vi "Percent-Decode String.vi"(10 "Pct-Encoded String":string) -> (2 "String":string)   [LabVIEW 2013, in "openURI.lvlib"]
uses:
  openURI.lvlib
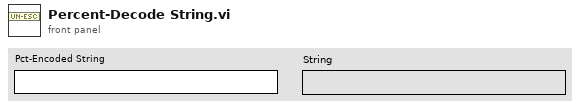
[diagram p1: front panel]
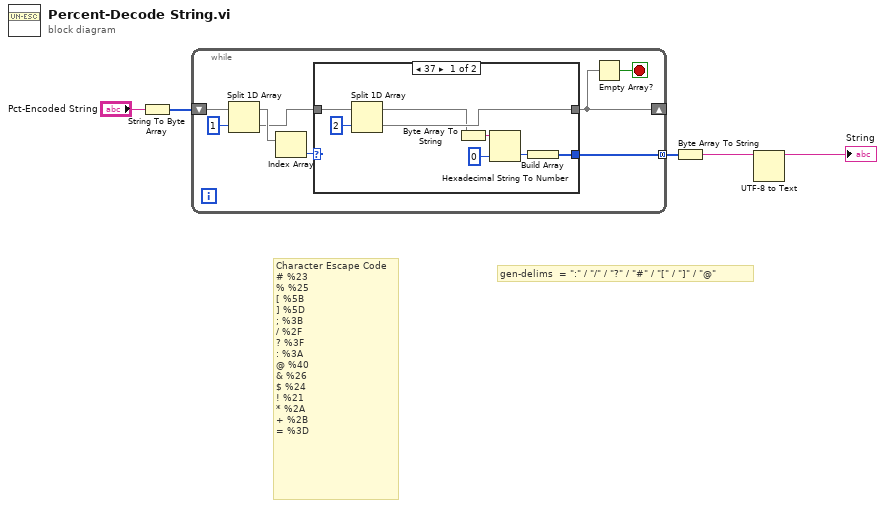
[diagram p0: block diagram]
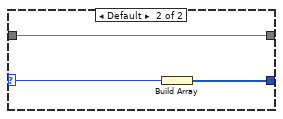
[diagram p2: hidden frame]
diagram:
  # "gen-delims  = \":\" / \"/\" / \"?\" / \"#\" / \"[\" / \"]\" / \"@\""
  # "Character\tEscape Code\n#\t%23\n%\t%25\n[\t%5B\n]\t%5D\n;\t%3B\n/\t%2F\n?\t%3F\n:\t%3A\n@\t%40\n&\t%26\n$\t%24\n!\t%21\n*\t%2A\n+\t%2B\n=\t%3D"
  n1 = String To Byte Array(string="Pct-Encoded String") -> (unsigned byte array=w5:u8[])
  n2 = while {
    shift-right: [w6] -> _
    shift-left: w5 -> [w13]
    tunnel: [w7] -> w4 mode=concatenating
    stop <- w10 stop-if-true
    n3 = Split 1D Array(array=w13, index=1) -> (first subarray=w11:u8[], second subarray=w8:u8[])
    n4 = Index Array(array=w11) -> (element=w9:u8)  [unwired: 1 in]
    n5 = case shown="37" w9 {
      selector: w9 -> [_ w23]
      tunnel: w8 -> [w20 w24]
      tunnel: [w19 w24] -> w6
      tunnel: [w15 w22] -> w7
      frame 37 {
        n6 = Split 1D Array(array=w20, index=2) -> (first subarray=w18:u8[], second subarray=w19:u8[])
        n7 = Byte Array To String(unsigned byte array=w18) -> (string=w17:string)
        n8 = Hexadecimal String To Number(string=w17, default (0uL)=u8 0 ("default (0 U32)")) -> (number=w16:u8)  [unwired: 1 in, 1 out]
        n9 = Build Array(w16) -> (w15:u8[])
      }
      frame Default {
        n10 = Build Array(w23) -> (w22:u8[])
      }
    }
    n11 = Empty Array?(array=w6) -> (empty?=w10:bool)
  }
  n12 = Byte Array To String(unsigned byte array=w4) -> (string=w2:string)
  n13 = UTF-8 to Text(11:w2) -> (3:→"String":string)  [unwired: 1 in, 1 out]
